vi "Set Timing Cfg.vi"(8 "error in":errorcluster, 9 "ReadBlk":i32, 10 "Rate":dbl, 11 "TimingGrp in":refnum<class "TimingGrp.lvclass">) -> (0 "error out":errorcluster, 3 "TimingGrp in":refnum<class "TimingGrp.lvclass">)   [LabVIEW 2012, in "Configuration Grandmaster.lvlib" / "TimingGrp.lvclass"]
uses:
  TimingGrp.lvclass
  TimingGrp.lvclass/TimingGrp.ctl
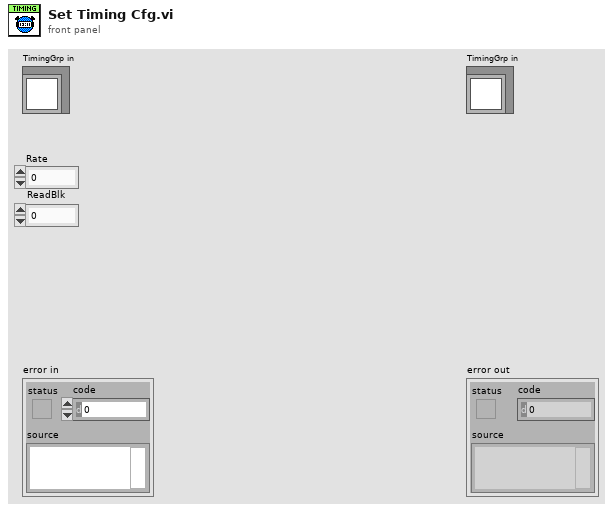
[diagram p1: front panel]
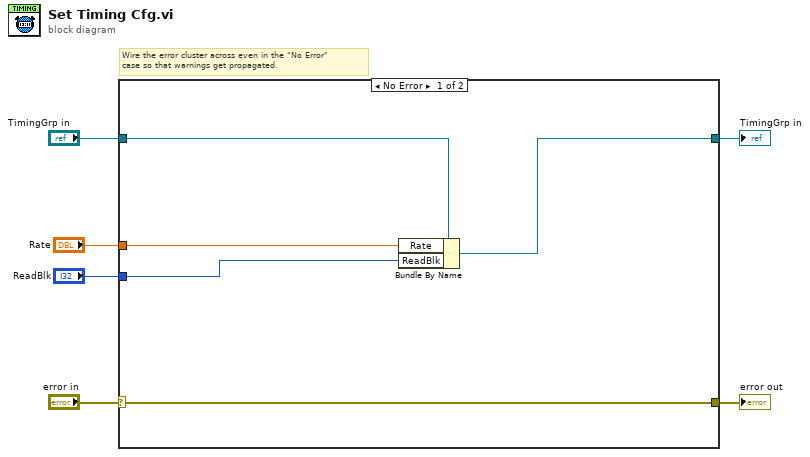
[diagram p0: block diagram]
diagram:
  # "Wire the error cluster across even in the \"No Error\"\ncase so that warnings get propagated."
  n1 = case shown="No Error" "error in" {
    selector: "error in" -> [w11 w13]
    tunnel: [w11 w13] -> w5
    tunnel: [w9 w12] -> w3
    tunnel: "TimingGrp in" -> [w10 w12]
    tunnel: "Rate" -> [w8 _]
    tunnel: "ReadBlk" -> [w7 _]
    frame No Error {
      n2 = Bundle By Name(cluster=w10, "Rate"=w8, "ReadBlk"=w7) -> (w9:refnum<class "TimingGrp.lvclass">)
    }
    frame Error {
    }
  }
  "error out" <- w5
  "TimingGrp in" <- w3
